vi "Module - RH_BELAJA.vi"() -> ()   [LabVIEW 2020]
uses:
  Control/State - eFGV.ctl
panel:
  out "Site Name":string="RH BELAJA (22.75 kWp)"
  out "BANK-02 Status 2":bool
  out "BANK-01 Status 2":bool
  out "BANK-02-TEMP 2":dbl caption="T_bat" format="%#_g °C"
  out "BANK-02-IDC 2":dbl caption="I_bat" format="%#_g A"
  out "BANK-02-VDC 2":dbl caption="V_bat" format="%#_g V"
  out "BANK-02-SOC 2":dbl caption="SOC" format="%#_g %"
  out "BANK-01-TEMP 2":dbl caption="T_bat" format="%#_g °C"
  out "BANK-01-IDC 2":dbl caption="I_bat" format="%#_g A"
  out "BANK-01-VDC 2":dbl caption="V_bat" format="%#_g V"
  out "BANK-01-SOC 2":dbl caption="SOC" format="%#_g %"
  out "SI-01 Status 4":bool
  out "SI-01-FREQ 4":dbl caption="FREQ" format="%.0f Hz"
  out "SI-01-L3 4":dbl caption="L3" format="%.0f V"
  out "SI-01-L2 4":dbl caption="L2" format="%.0f V"
  out "SI-01-L1 4":dbl caption="L1" format="%.0f V"
  out "SI-01-PAC 4":dbl caption="Pac" format="%.0f W"
  out "SI-01 Status 3":bool
  out "SI-M Status 2":bool
  out "SI-01-FREQ 3":dbl caption="FREQ" format="%.0f Hz"
  out "SI-01-L3 3":dbl caption="L3" format="%.0f V"
  out "SI-01-L2 3":dbl caption="L2" format="%.0f V"
  out "SI-01-L1 3":dbl caption="L1" format="%.0f V"
  out "SI-01-PAC 3":dbl caption="Pac" format="%.0f W"
  out "SI-M-FREQ 2":dbl caption="FREQ" format="%.0f Hz"
  out "SI-M-L3 2":dbl caption="L3" format="%.0f V"
  out "SI-M-L2 2":dbl caption="L2" format="%.0f V"
  out "SI-M-L1 2":dbl caption="L1" format="%.0f V"
  out "SI-M-PAC 2":dbl caption="Pac" format="%.0f W"
  out "SB-02 Status 2":bool
  out "SB-02-B-IAC 2":dbl caption="B.Idc" format="%.0f A"
  out "SB-02-B-VAC 2":dbl caption="B.Vdc" format="%.0f V"
  out "SB-02-A-IAC 2":dbl caption="A.Idc" format="%.0f A"
  out "SB-02-A-VAC 2":dbl caption="A.Vdc" format="%.0f V"
  out "SB-02-PAC 2":dbl caption="Pac" format="%#_g W"
  out "SI-01 Status 2":bool
  out "SI-01-FREQ 2":dbl caption="FREQ" format="%.0f Hz"
  out "SI-01-L3 2":dbl caption="L3" format="%.0f V"
  out "SI-01-L2 2":dbl caption="L2" format="%.0f V"
  out "SI-01-L1 2":dbl caption="L1" format="%.0f V"
  out "SI-01-PAC 2":dbl caption="Pac" format="%.0f W"
  out "PM-01 Status":bool
  out "SI-01 Status":bool
  out "SI-M Status":bool
  out "BANK-02 Status":bool
  out "BANK-01 Status":bool
  out "SB-02 Status":bool
  out "SB-01 Status":bool
  out "SI-01-FREQ":dbl caption="FREQ" format="%.0f Hz"
  out "SI-01-L3":dbl caption="L3" format="%.0f V"
  out "SI-01-L2":dbl caption="L2" format="%.0f V"
  out "SI-01-L1":dbl caption="L1" format="%.0f V"
  out "SI-01-PAC":dbl caption="Pac" format="%.0f W"
  out "BANK-02-TEMP":dbl caption="T_bat" format="%#_g °C"
  out "BANK-02-IDC":dbl caption="I_bat" format="%#_g A"
  out "BANK-02-VDC":dbl caption="V_bat" format="%#_g V"
  out "BANK-02-SOC":dbl caption="SOC" format="%#_g %"
  out "SB-02-B-IAC":dbl caption="B.Idc" format="%.0f A"
  out "SB-02-B-VAC":dbl caption="B.Vdc" format="%.0f V"
  out "SB-02-A-IAC":dbl caption="A.Idc" format="%.0f A"
  out "SB-02-A-VAC":dbl caption="A.Vdc" format="%.0f V"
  out "SB-02-PAC":dbl caption="Pac" format="%#_g W"
  out "PM-01-FREQ":dbl caption="Freq" format="%.0f Hz"
  out "PM-01-IAC":dbl caption="Iac" format="%.0f A"
  out "PM-01-VAC":dbl caption="Vac" format="%.0f V"
  out "PM-01-PAC":dbl caption="Pac" format="%.0f W"
  out "SI-M-FREQ":dbl caption="FREQ" format="%.0f Hz"
  out "SI-M-L3":dbl caption="L3" format="%.0f V"
  out "SI-M-L2":dbl caption="L2" format="%.0f V"
  out "SI-M-L1":dbl caption="L1" format="%.0f V"
  out "SI-M-PAC":dbl caption="Pac" format="%.0f W"
  out "BANK-01-TEMP":dbl caption="T_bat" format="%#_g °C"
  out "BANK-01-IDC":dbl caption="I_bat" format="%#_g A"
  out "BANK-01-VDC":dbl caption="V_bat" format="%#_g V"
  out "BANK-01-SOC":dbl caption="SOC" format="%#_g %"
  out "SB-01-B-IAC":dbl caption="B.Idc" format="%.0f A"
  out "SB-01-B-VAC":dbl caption="B.Vdc" format="%.0f V"
  out "SB-01-A-IAC":dbl caption="A.Idc" format="%.0f A"
  out "SB-01-A-VAC":dbl caption="A.Vdc" format="%.0f V"
  out "SB-01-PAC":dbl caption="Pac" format="%.0f W"
  # "BANK-1"
  # "STP1"
  # "STP2"
  # "BANK-2"
  # "BANK-1"
  # "BANK-2"
  # "SI-M"
  # "SI-M"
  # "SI-01"
  # "SI-01"
  # "SI-01"
  # "SI-01"
  # "STP3"
  # "PM-01"
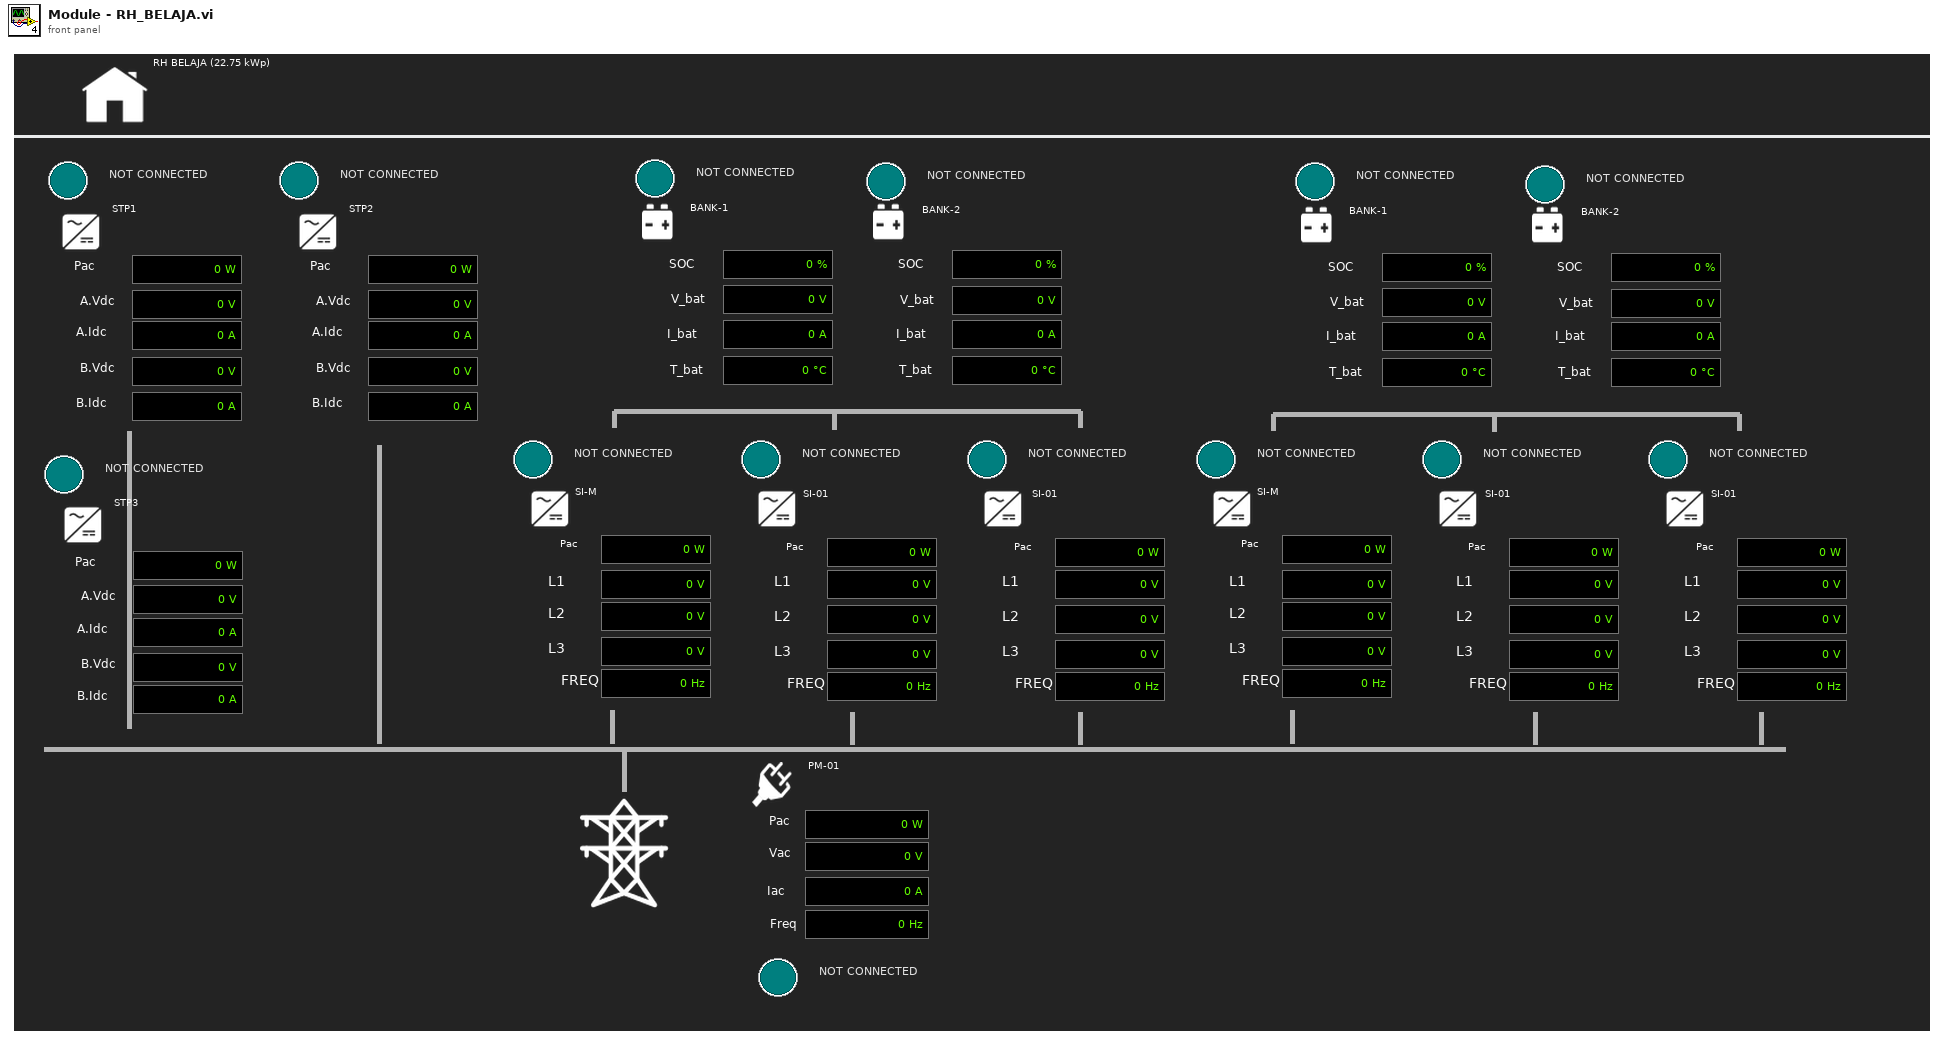
[diagram p1: front panel]
types:
  T1 = typedef "State - eFGV.ctl" = enum16{"Init", "Read", "Write", "Close"}
  T2 = typedef "Device Name.ctl" = enum16{"SB-01", "SB-02", "BANK-01", "BANK-02", "SI-M", "SI-01", "PM-01"}
  T3 = typedef "Data Struct - SB.ctl" = cluster{"Pac":dbl, "A.Vdc":dbl, "A.Idc":dbl, "B.Vdc":dbl, "B.Idc":dbl}
  T4 = typedef "Data Struct - Bank.ctl" = cluster{"SOC":dbl, "V_Bat":dbl, "I_Bat":dbl, "T_Bat":dbl}
  T5 = typedef "Data Struct - SI.ctl" = cluster{"Pac":dbl, "L1":dbl, "L2":dbl, "L3":dbl, "Freq":dbl}
  T6 = typedef "Data Struct - PM.ctl" = cluster{"Pac":dbl, "Vac":dbl, "Iac":dbl, "Freq":dbl}
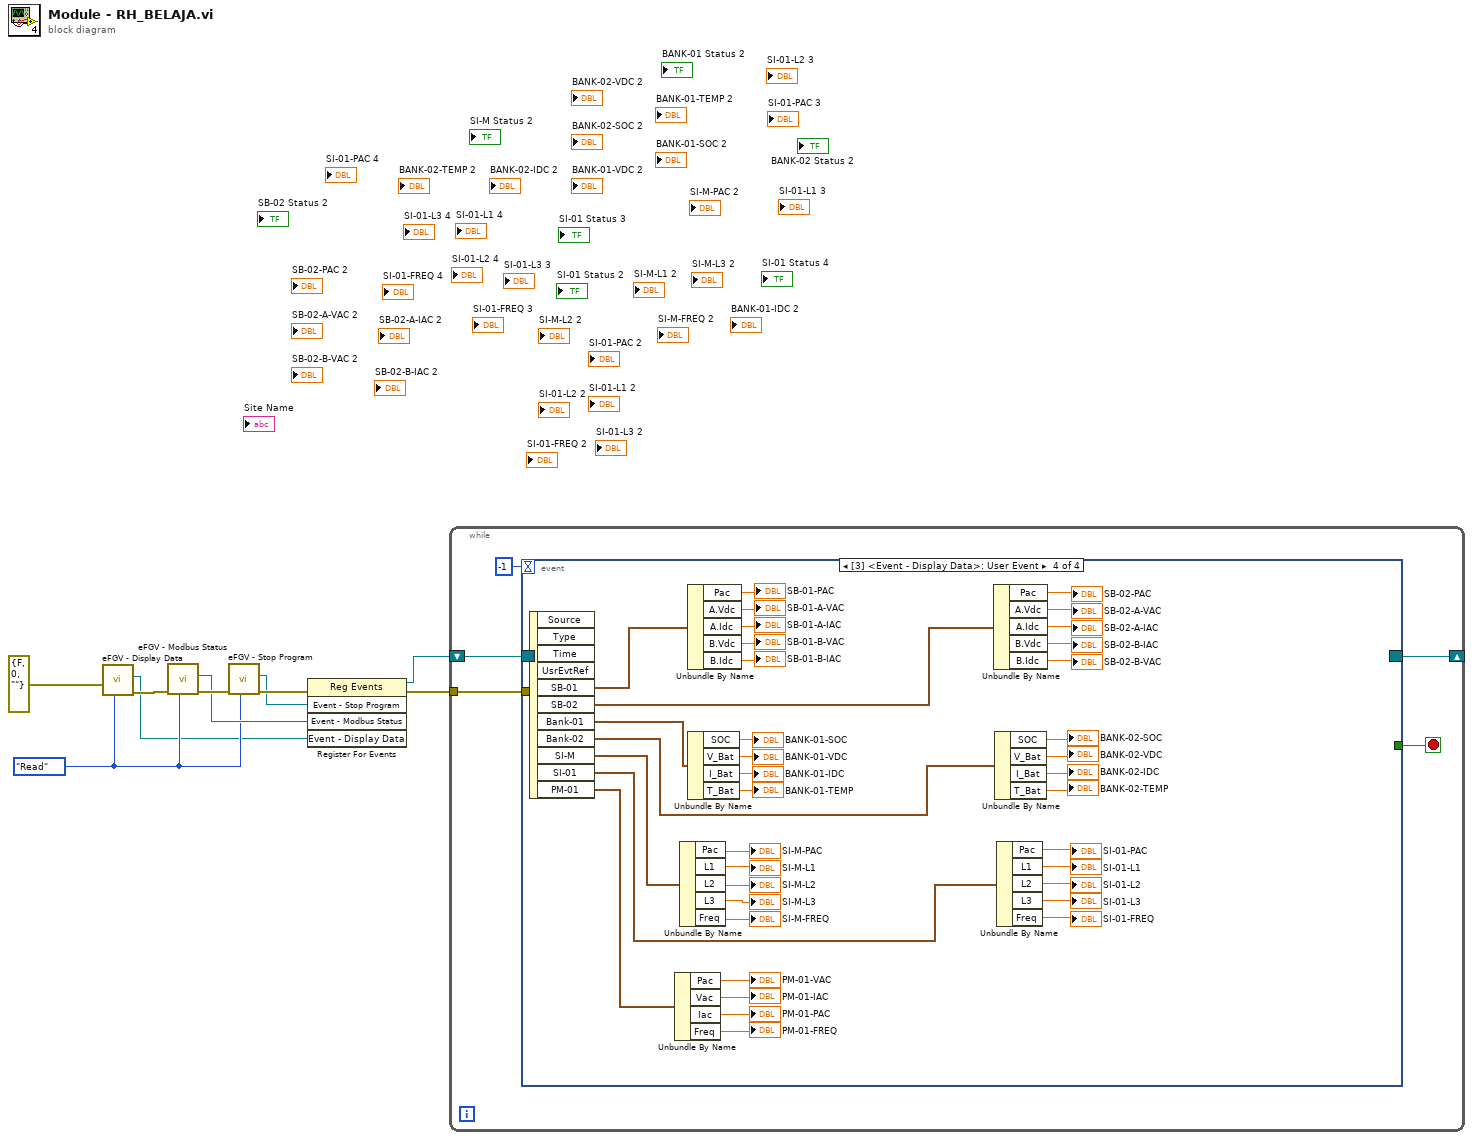
[diagram p0: block diagram]
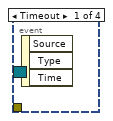
[diagram p2: hidden frame]
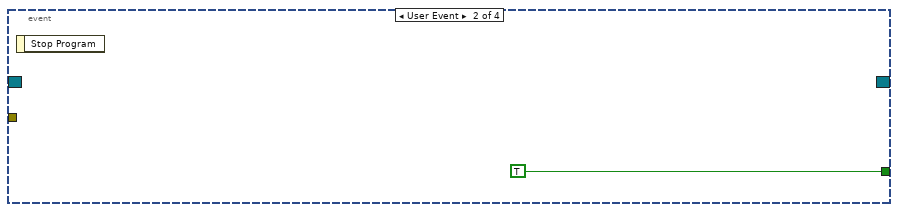
[diagram p3: hidden frame]
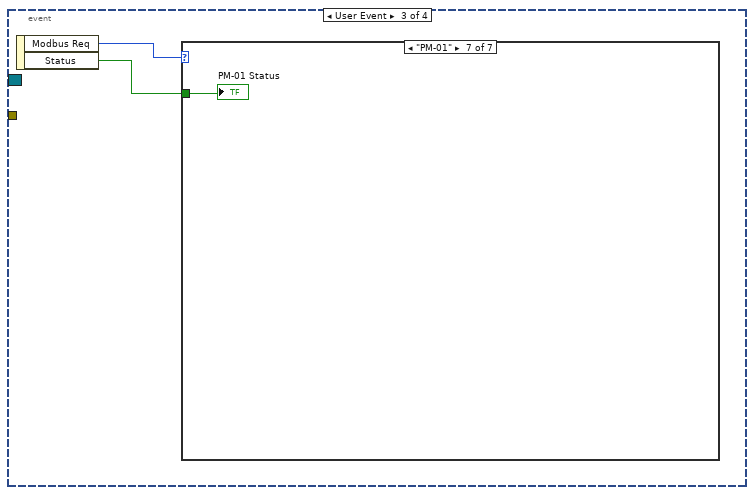
[diagram p4: hidden frame]
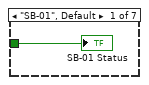
[diagram p5: hidden frame]
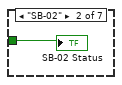
[diagram p6: hidden frame]
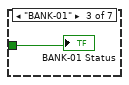
[diagram p7: hidden frame]
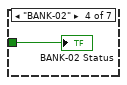
[diagram p8: hidden frame]
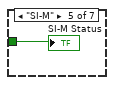
[diagram p9: hidden frame]
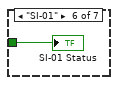
[diagram p10: hidden frame]
diagram:
  w2 = State_-_eFGV."Read" ("State - eFGV")
  n1 = call "eFGV - Display Data.vi"("State - eFGV"=w2, "error in (no error)"=errorcluster {"status"=FALSE, "code"=0, "source"=""}) -> ("error out"=w4:errorcluster, "Event - Display Data"=w1:refnum<user-event>)  [unwired: 8 in]
  n2 = call "eFGV - Modbus Status.vi"("State - eFGV"=w2, "error in (no error)"=w4) -> ("error out"=w6:errorcluster, "Event - Modbus Status"=w5:refnum<user-event>)  [unwired: 8 in]
  n3 = call "eFGV - Stop Program.vi"("State - eFGV"=w2, "error in (no error)"=w6) -> ("error out"=w9:errorcluster, "Event - Stop Program"=w8:refnum<user-event>)  [unwired: 8 in]
  n4 = register-events(error in=w9, w8, w5, w1) -> (reference out=w7:refnum<event-registration>, error out=w10:errorcluster)  [unwired: 1 in]
  n5 = while {
    tunnel: w10 -> [w14]
    shift-right: [w13] -> _
    shift-left: w7 -> [w15]
    stop <- w12 stop-if-true
    n6 = event shown="[3] <Event - Display Data>: User Event" {
      selector: w15 -> [_ _ _ _]
      dyn-events: [_ _ _ _] -> w13
      timeout: -1 -> [_ _ _ _]
      tunnel: w14 -> [_ _ _ _]
      tunnel: [_ TRUE _ _] -> w12
      event Timeout {
        n7 = event-data() -> ()  [unwired: 1 in, 3 out]
      }
      event User Event {
        n8 = event-data() -> ()  [unwired: 1 in, 1 out]
      }
      event User Event {
        n9 = event-data() -> ("Modbus Req"=w18:T2, "Status"=w17:bool)  [unwired: 1 in]
        n10 = case shown="\"PM-01\"" w18 {
          tunnel: w17 -> [w19 w20 w21 w22 w23 w24 w25]
          frame "SB-01", Default {
            "SB-01 Status" <- w19
          }
          frame "SB-02" {
            "SB-02 Status" <- w20
          }
          frame "BANK-01" {
            "BANK-01 Status" <- w21
          }
          frame "BANK-02" {
            "BANK-02 Status" <- w22
          }
          frame "SI-M" {
            "SI-M Status" <- w23
          }
          frame "SI-01" {
            "SI-01 Status" <- w24
          }
          frame "PM-01" {
            "PM-01 Status" <- w25
          }
        }
      }
      event User Event {
        n11 = event-data() -> ("SB-01"=w64:T3, "SB-02"=w63:T3, "Bank-01"=w52:T4, "Bank-02"=w51:T4, "SI-M"=w42:T5, "SI-01"=w36:T5, "PM-01"=w30:T6)  [unwired: 1 in, 4 out]
        n12 = Unbundle By Name(w30) -> ("Pac"=→"PM-01-VAC":dbl, "Vac"=→"PM-01-IAC":dbl, "Iac"=→"PM-01-PAC":dbl, "Freq"=→"PM-01-FREQ":dbl)
        n13 = Unbundle By Name(w42) -> ("Pac"=→"SI-M-PAC":dbl, "L1"=→"SI-M-L1":dbl, "L2"=→"SI-M-L2":dbl, "L3"=→"SI-M-L3":dbl, "Freq"=→"SI-M-FREQ":dbl)
        n14 = Unbundle By Name(w64) -> ("Pac"=→"SB-01-PAC":dbl, "A.Vdc"=→"SB-01-A-VAC":dbl, "A.Idc"=→"SB-01-A-IAC":dbl, "B.Vdc"=→"SB-01-B-VAC":dbl, "B.Idc"=→"SB-01-B-IAC":dbl)
        n15 = Unbundle By Name(w52) -> ("SOC"=→"BANK-01-SOC":dbl, "V_Bat"=→"BANK-01-VDC":dbl, "I_Bat"=→"BANK-01-IDC":dbl, "T_Bat"=→"BANK-01-TEMP":dbl)
        n16 = Unbundle By Name(w63) -> ("Pac"=→"SB-02-PAC":dbl, "A.Vdc"=→"SB-02-A-VAC":dbl, "A.Idc"=→"SB-02-A-IAC":dbl, "B.Vdc"=→"SB-02-B-IAC":dbl, "B.Idc"=→"SB-02-B-VAC":dbl)
        n17 = Unbundle By Name(w51) -> ("SOC"=→"BANK-02-SOC":dbl, "V_Bat"=→"BANK-02-VDC":dbl, "I_Bat"=→"BANK-02-IDC":dbl, "T_Bat"=→"BANK-02-TEMP":dbl)
        n18 = Unbundle By Name(w36) -> ("Pac"=→"SI-01-PAC":dbl, "L1"=→"SI-01-L1":dbl, "L2"=→"SI-01-L2":dbl, "L3"=→"SI-01-L3":dbl, "Freq"=→"SI-01-FREQ":dbl)
      }
    }
  }
